vi "number1-state machine.vi"() -> ()   [LabVIEW 2014]
panel:
  in  "OK Button":bool
  in  "#s":dbl=10000.0 format="%0.2p"
  in  "Fs":dbl=1000.0 format="%0.2p"
  out "Logined":bool
  in  "stop":bool
  out "array":bool[](array[boolean])
  in  "Button":T1
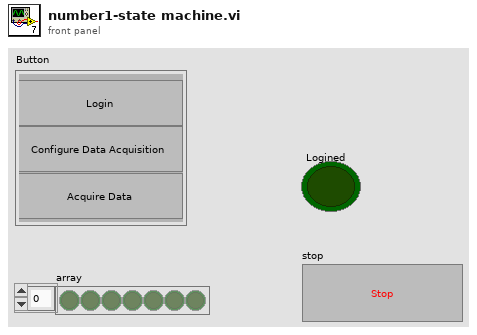
[diagram p1: front panel]
types:
  T1 = cluster{"OK Button":bool, "OK Button 2":bool, "OK Button 3":bool}
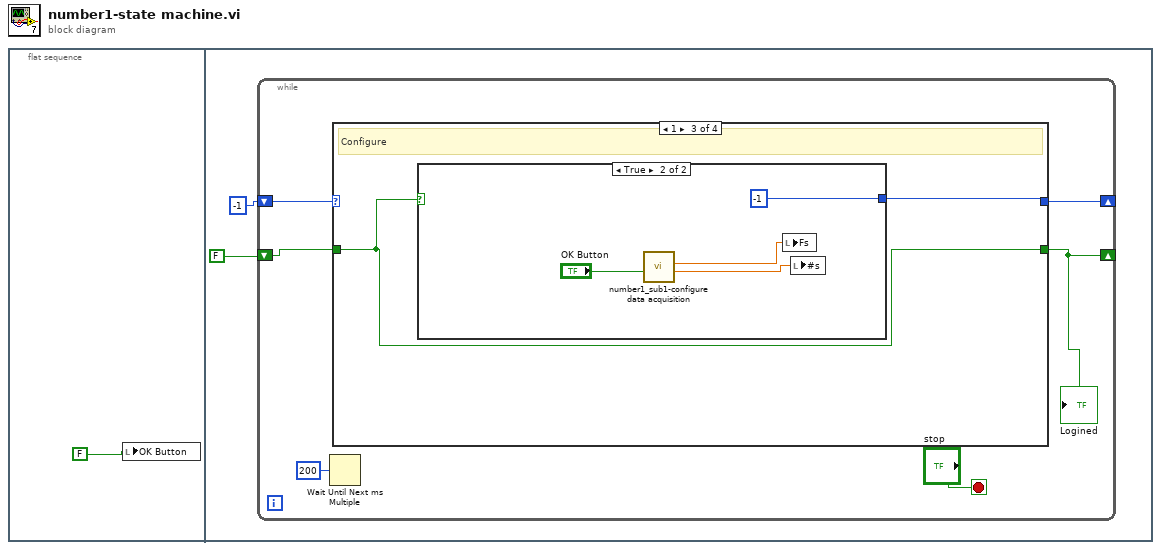
[diagram p0: block diagram]
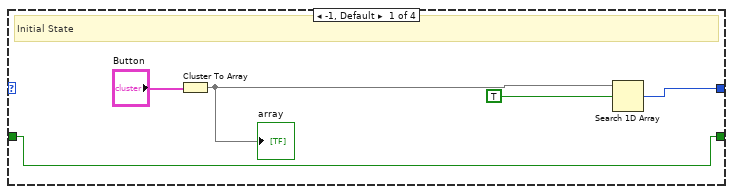
[diagram p2: hidden frame]
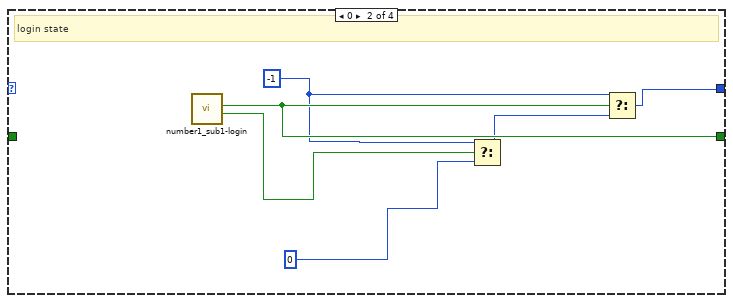
[diagram p3: hidden frame]
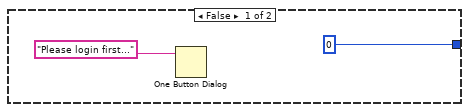
[diagram p4: hidden frame]
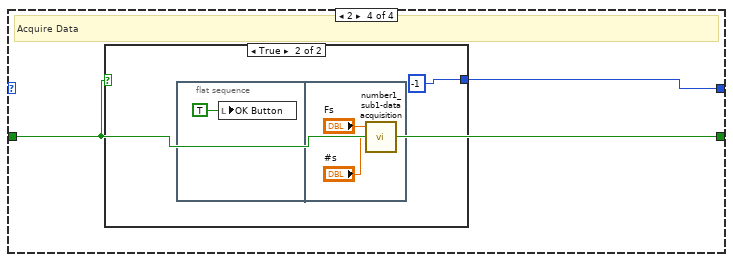
[diagram p5: hidden frame]
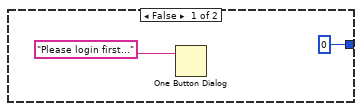
[diagram p6: hidden frame]
diagram:
  n1 = flat-sequence {
    frame #0 {
      n2 = local write "OK Button"(FALSE ("OK Button")) -> ()
    }
    frame #1 {
      n3 = while {
        shift-right: [w8] -> _
        shift-left: -1 -> [w9]
        shift-right: [w7] -> _
        shift-left: FALSE -> [w6]
        stop <- "stop" stop-if-true
        n4 = Wait Until Next ms Multiple(millisecond multiple=u32 200) -> ()  [unwired: 1 out]
        n5 = case shown="1" w9 {
          tunnel: [w11 w19 w21 w29] -> w8
          tunnel: [w10 w20 w22 w30] -> w7
          tunnel: w6 -> [w10 _ w22 w30]
          frame -1, Default {
            # "Initial State"
            n6 = Cluster To Array(cluster="Button") -> (array=w13:bool[])
            "array" <- w13
            n7 = Search 1D Array(1D array=w13, element=TRUE) -> (index of element=w11:i32)  [unwired: 1 in]
          }
          frame 0 {
            w17 = -1
            # "login state"
            n8 = call "number1_sub1-login.vi"() -> ("UserCancelled"=w18:bool, "Correct"=w20:bool)  [unwired: 10 in]
            n9 = Select(t=w17, s=w18, f=0) -> (s? t:f=w15:i32)
            n10 = Select(t=w17, s=w20, f=w15) -> (s? t:f=w19:i32)
          }
          frame 1 {
            # "Configure"
            n11 = case shown="True" w22 {
              tunnel: [0 -1] -> w21
              frame False {
                n12 = One Button Dialog(message="Please login first...") -> ()  [unwired: 1 in, 1 out]
              }
              frame True {
                n13 = call "number1_sub1-configure data acquisition.vi"("OK Button"="OK Button") -> ("samples per acquisition 2"=w26:dbl, "sampling rate (samples/sec) 2"=w27:dbl)  [unwired: 5 in]
                n14 = local write "Fs"(w27) -> ()
                n15 = local write "#s"(w26) -> ()
              }
            }
          }
          frame 2 {
            # "Acquire Data"
            n16 = case shown="True" w30 {
              tunnel: [0 -1 ("index of element")] -> w29
              frame False {
                n17 = One Button Dialog(message="Please login first...") -> ()  [unwired: 1 in, 1 out]
              }
              frame True {
                n18 = flat-sequence {
                  frame #0 {
                    n19 = local write "OK Button"(TRUE ("OK Button")) -> ()
                  }
                  frame #1 {
                    n20 = call "number1_sub1-data acquisition.vi"("#s"="#s", "Fs"="Fs") -> ()  [unwired: 3 in, 1 out]
                  }
                }
              }
            }
          }
        }
        "Logined" <- w7
      }
    }
  }
